vi "Actor Core.vi"(8 "error in":errorcluster, 11 "Nested in":refnum<class "Stage Controller.lvclass">) -> (0 "error out":errorcluster, 3 "Actor out":refnum<class "Actor.lvclass">)   [LabVIEW 2020, in "Stage.lvlib" / "Stage Controller.lvlib" / "Stage Controller.lvclass"]
doc: "(<B>Filename</B>: Actor Framework.lvlib:Actor.lvclass:Actor Core.vi)\n\nReceives messages to the actor, reacts to them, and initiates any error handling that may shut the actor down.\n\nDescendant classes may override this VI to append parallel tasks for the actor to complete while it handles messages. Overrides use the Call Parent Method node."
uses:
  Stage Controller.lvclass
  C:/Program Files/National Instruments/LabVIEW 2020/vi.lib/ActorFramework/Actor/Actor.lvclass
  <vilib>/ActorFramework/Actor/Actor.lvclass
  Stage Controller.lvclass/Stage Controller.ctl
  <vilib>/ActorFramework/Actor/Actor.lvclass/Actor.ctl
  <vilib>/ActorFramework/Message Enqueuer/Message Enqueuer.lvclass/Message Enqueuer.ctl
  HAL Layer/Stage/Stage Messages/SetRelativePositionUm Msg/SetRelativePositionUm Msg.lvclass/SetRelativePositionUm Msg.ctl
  HAL Layer/Stage/Stage Messages/SetPositionUm Msg/SetPositionUm Msg.lvclass/SetPositionUm Msg.ctl
  HAL Layer/Stage/Stage Messages/Set Acquisition Interval Msg/Set Acquisition Interval Msg.lvclass/Set Acquisition Interval Msg.ctl
  <vilib>/ActorFramework/Message Enqueuer/Init from Existing Queue.vi
  <vilib>/ActorFramework/Message Enqueuer/Enqueue.vi
  HAL Layer/Stage/Stage Messages/SetRelativePositionUm Msg/SetRelativePositionUm Msg.lvclass
  C:/Program Files/National Instruments/LabVIEW 2020/vi.lib/ActorFramework/Message/Message.lvclass
  HAL Layer/Stage/Stage Messages/SetPositionUm Msg/SetPositionUm Msg.lvclass
  HAL Layer/Stage/Stage Messages/Set Acquisition Interval Msg/Set Acquisition Interval Msg.lvclass
  <vilib>/ActorFramework/Stop Msg/Stop Msg.lvclass
  <vilib>/ActorFramework/Message Priority Queue/Priority Enqueue.vi
  <vilib>/ActorFramework/Message Enqueuer/Message Enqueuer.lvclass
panel:
  in  "Interval(ms)":dbl min=0.0 max=200.0
  in  "Stop Button":bool
  in  "StageZ":dbl min=0.0 max=200.0
  in  "StageY":dbl min=0.0 max=200.0
  in  "StageX":dbl min=0.0 max=200.0
  out "NanoStage X":dbl(graph)
  out "NanoStage  Y":dbl(graph)
  out "NanoStage Z":dbl(graph)
  in  "ZIncreatement+":dbl min=0.0 max=50.0
  in  "ZIncreatement++":dbl min=0.0 max=50.0
  in  "StageX-":bool
  in  "StageX+":bool
  in  "StageY+":bool
  in  "StageY-":bool
  in  "StageY++":bool
  in  "StageX--":bool
  in  "StageX++":bool
  in  "StageY--":bool
  in  "XYIncreatement+":dbl min=0.0 max=50.0
  in  "XYIncreatement++":dbl min=0.0 max=100.0
  in  "StageZ++":bool
  in  "StageZ--":bool
  in  "StageZ+":bool
  in  "StageZ-":bool
  # "Inc.(μm)"
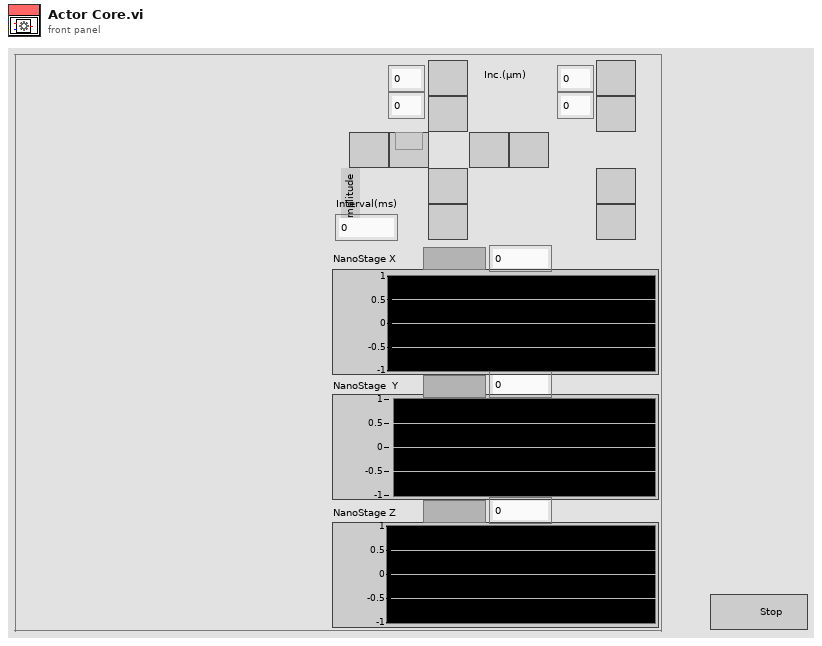
[diagram p1: front panel]
types:
  T1 = cluster{"Stop":refnum<user-event>, "NanoStage X":refnum<user-event>, "NanoStage  Y":refnum<user-event>, "NanoStage Z":refnum<user-event>}
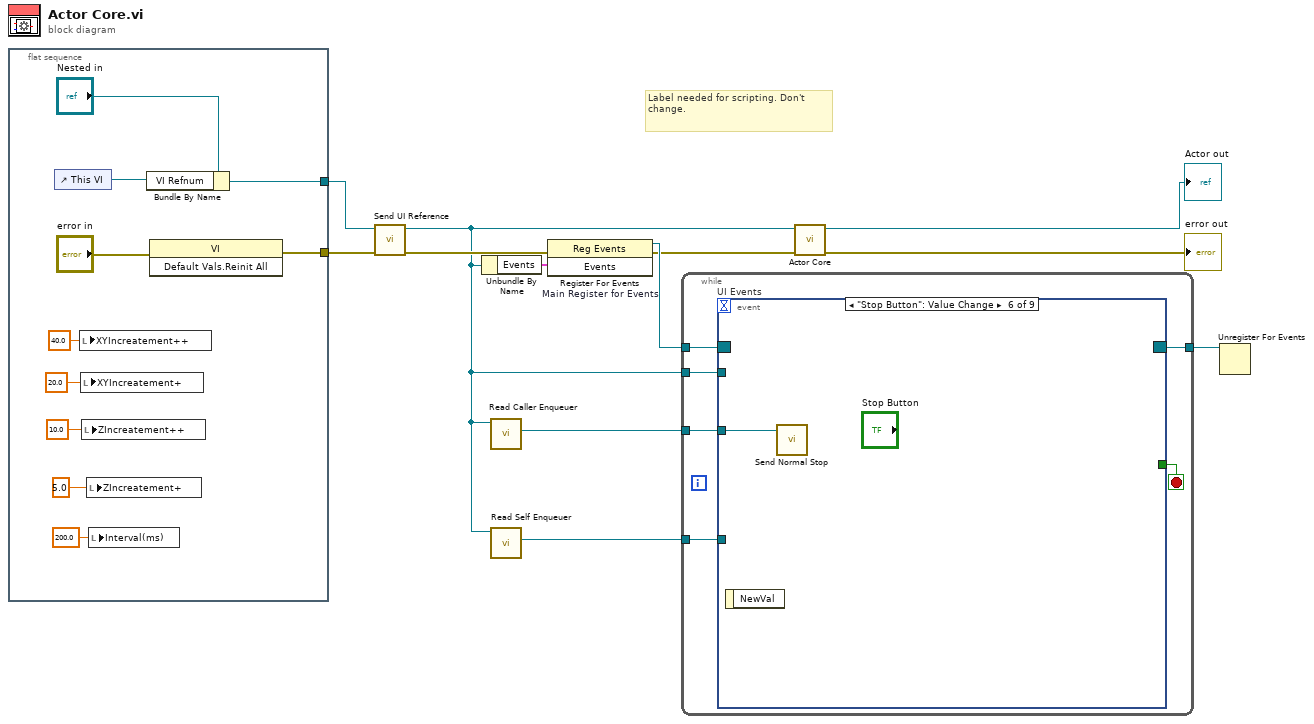
[diagram p0: block diagram]
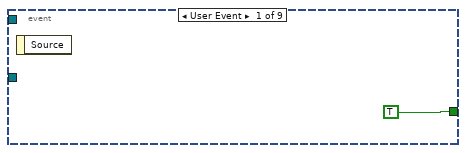
[diagram p2: hidden frame]
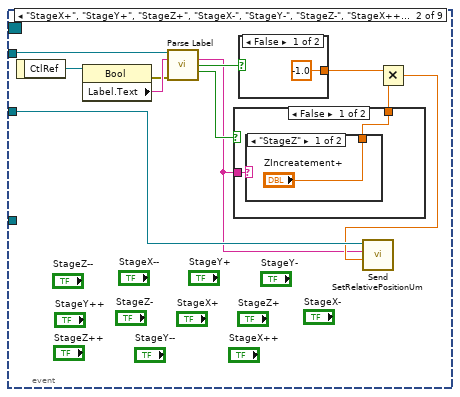
[diagram p3: hidden frame]
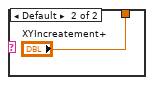
[diagram p4: hidden frame]
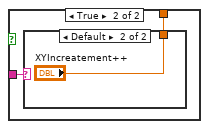
[diagram p5: hidden frame]
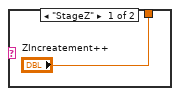
[diagram p6: hidden frame]
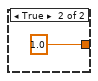
[diagram p7: hidden frame]
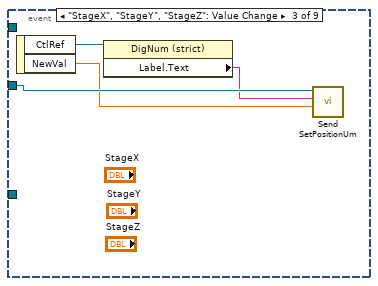
[diagram p8: hidden frame]
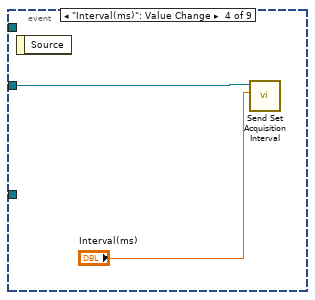
[diagram p9: hidden frame]
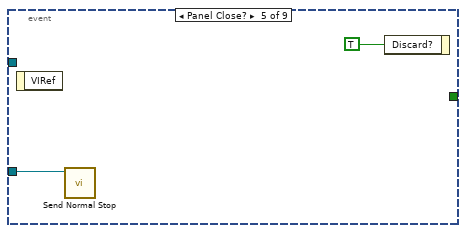
[diagram p10: hidden frame]
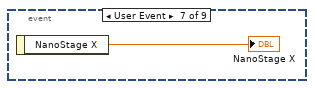
[diagram p11: hidden frame]
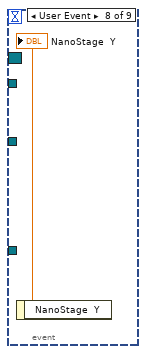
[diagram p12: hidden frame]
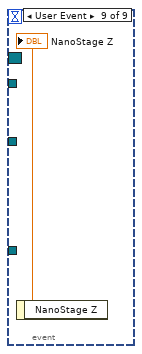
[diagram p13: hidden frame]
diagram:
  # "Label needed for scripting. Don't change."
  n1 = flat-sequence {
    tunnel: [w20] -> w5
    tunnel: [w19] -> w4
    frame #0 {
      n2 = control-ref of="This VI"() -> (w18:refnum<vi>)
      n3 = local write "XYIncreatement++"(40.0 ("XYIncreatement++")) -> ()
      n4 = local write "XYIncreatement+"(20.0 ("XYIncreatement++")) -> ()
      n5 = local write "ZIncreatement++"(10.0 ("XYIncreatement++")) -> ()
      n6 = local write "ZIncreatement+"(5.0 ("XYIncreatement++")) -> ()
      n7 = local write "Interval(ms)"(200.0 ("Interval(ms)")) -> ()
      n8 = Bundle By Name(cluster="Nested in", "VI Refnum"=w18) -> (w20:refnum<class "Stage Controller.lvclass">)
      n9 = invoke class="VI" method="Default Vals.Reinit All"(error in="error in") -> (error out=w19:errorcluster)  [unwired: 2 in, 2 out]
    }
  }
  n10 = call-dynamic "Send UI Reference.vi"("error in (no error)"=w4, "Stage Controller in"=w5) -> ("error out"=w3:errorcluster, "Stage Controller out"=w2:refnum<class "Stage Controller.lvclass">)  [unwired: 8 in]
  n11 = Unbundle By Name(w2) -> ("Events"=w9:T1)
  n12 = call <vilib>:"Read Caller Enqueuer.vi"("Actor"=w2) -> ("Caller Enqueuer"=w1:refnum<class "Message Enqueuer.lvclass">)  [unwired: 10 in]
  n13 = call <vilib>:"Read Self Enqueuer.vi"("Actor"=w2) -> ("Self Enqueuer"=w7:refnum<class "Message Enqueuer.lvclass">)  [unwired: 10 in]
  n14 = register-events "Main Register for Events"(error in=w3, w9) -> (reference out=w10:refnum<event-registration>, error out=w6:errorcluster)  [unwired: 1 in]
  n15 = while {
    tunnel: w10 -> [w28]
    tunnel: [w26] -> w8
    tunnel: w7 -> [w25]
    tunnel: w2 -> [w24]
    tunnel: w1 -> [w23]
    stop <- w27 stop-if-true
    n16 = event "UI Events" shown="[5] \"Stop Button\": Value Change" {
      selector: w28 -> [_ _ _ _ _ _ _ _ _]
      dyn-events: [_ _ _ _ _ _ _ _ _] -> w26
      timeout: _ -> [_ _ _ _ _ _ _ _ _]
      tunnel: [TRUE _ _ _ _ _ _ _ _] -> w27
      tunnel: w25 -> [_ _ _ _ w57 _ _ _ _]
      tunnel: w24 -> [_ w37 _ _ _ _ _ _ _]
      tunnel: w23 -> [_ w36 w53 w56 _ w59 _ _ _]
      event User Event {
        n17 = event-data() -> ()  [unwired: 1 in, 1 out]
      }
      event "StageX+", "StageY+", "StageZ+", "StageX-", "StageY-", "StageZ-", "StageX++", "StageY++", "StageZ++", "StageX--", "StageY--", "StageZ--": Value Change {
        n18 = event-data() -> ("CtlRef"=w40:refnum<vi>)  [unwired: 1 in]
        n19 = property class="Bool"(reference=w40) -> (error out=w38:errorcluster, "Label.Text"=w39:string)  [unwired: 1 in, 1 out]
        n20 = call-dynamic "Parse Label.vi"("Stage Controller in"=w37, "Label.Text"=w39, "error in (no error)"=w38) -> ("Stage Label"=w30:string, "Increase?"=w35:bool, "Big Step?"=w34:bool)  [unwired: 8 in, 2 out]
        n21 = case shown="False" w34 {
          tunnel: [w42 w46] -> w32
          tunnel: w30 -> [w41 w45]
          frame False {
            n22 = case shown="\"StageZ\"" w41 {
              tunnel: ["ZIncreatement+" "XYIncreatement+"] -> w42
              frame "StageZ" {
              }
              frame Default {
              }
            }
          }
          frame True {
            n23 = case shown="Default" w45 {
              tunnel: ["ZIncreatement++" "XYIncreatement++"] -> w46
              frame "StageZ" {
              }
              frame Default {
              }
            }
          }
        }
        n24 = case shown="False" w35 {
          tunnel: [-1.0 ("XYIncreatement+") 1.0 ("XYIncreatement+")] -> w33
          frame False {
          }
          frame True {
          }
        }
        n25 = Multiply(x=w33, y=w32) -> (x*y=w31:dbl)
        n26 = call "Send SetRelativePositionUm.vi"("RelativeMoveum"=w31, "Stage Label"=w30, "Message Enqueuer"=w36) -> ()  [unwired: 7 in, 2 out]
      }
      event "StageX", "StageY", "StageZ": Value Change {
        n27 = event-data() -> ("CtlRef"=w54:refnum<vi>, "NewVal"=w51:dbl)  [unwired: 1 in]
        n28 = property class="DigNum (strict)"(reference=w54) -> ("Label.Text"=w52:string)  [unwired: 1 in, 2 out]
        n29 = call "Send SetPositionUm.vi"("Positionum"=w51, "Stage Label"=w52, "Message Enqueuer"=w53) -> ()  [unwired: 7 in, 2 out]
      }
      event "Interval(ms)": Value Change {
        n30 = event-data() -> ()  [unwired: 1 in, 1 out]
        n31 = call "Send Set Acquisition Interval.vi"("Interval(ms)"="Interval(ms)", "Message Enqueuer"=w56) -> ()  [unwired: 8 in, 2 out]
      }
      event Panel Close? {
        n32 = event-data() -> ()  [unwired: 1 in, 1 out]
        n33 = call <vilib>:"Send Normal Stop.vi"("Message Enqueuer"=w57) -> ()  [unwired: 10 in, 1 out]
        n34 = event-data("Discard?"=TRUE) -> ()  [unwired: 1 in, 1 out]
      }
      event "Stop Button": Value Change {
        n35 = event-data() -> ()  [unwired: 1 in, 1 out]
        n36 = call <vilib>:"Send Normal Stop.vi"("Message Enqueuer"=w59) -> ()  [unwired: 10 in, 1 out]
      }
      event User Event {
        n37 = event-data() -> ("NanoStage X"=→"NanoStage X":dbl)  [unwired: 1 in]
      }
      event User Event {
        n38 = event-data() -> ("NanoStage  Y"=→"NanoStage  Y":dbl)  [unwired: 1 in]
      }
      event User Event {
        n39 = event-data() -> ("NanoStage Z"=→"NanoStage Z":dbl)  [unwired: 1 in]
      }
    }
  }
  n40 = call-parent "Actor Core.vi"("error in"=w6, "Actor in"=w2) -> ("error out"=→"error out":errorcluster, "Actor out"=→"Actor out":refnum<class "Actor.lvclass">)  [unwired: 8 in]
  n41 = Unregister For Events(event registration refnum=w8) -> ()  [unwired: 1 in, 1 out]
